vi "getHighlightedRows.vi"(8 "error in (no error)":errorcluster, 11 "OutcomeList in":refnum<class "GoalList.lvclass">) -> (0 "error out":errorcluster, 2 "Highlighted Rows":i32[](array[numeric]), 3 "OutcomeList out":refnum<class "GoalList.lvclass">)   [LabVIEW 2020, in "GoalList.lvclass"]
uses:
  GoalList.lvclass
  Goal/Goal.lvclass
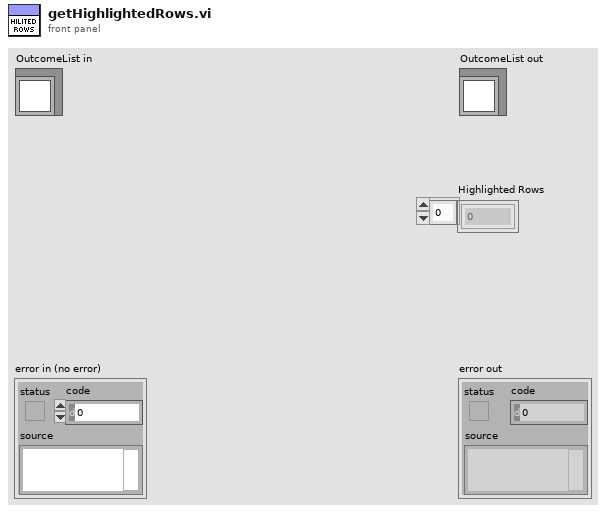
[diagram p1: front panel]
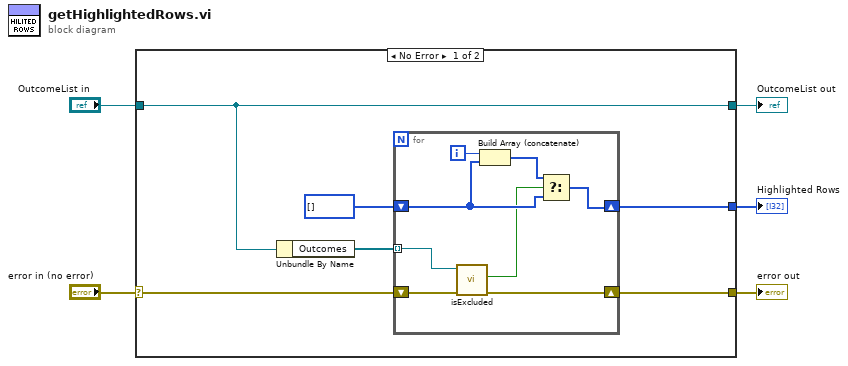
[diagram p0: block diagram]
diagram:
  n1 = case shown="No Error" "error in (no error)" {
    selector: "error in (no error)" -> [w8 w21]
    tunnel: [w7 w21] -> w4
    tunnel: [w9 w20] -> w2
    tunnel: "OutcomeList in" -> [w9 w20]
    tunnel: [w6 _] -> w1
    frame No Error {
      n2 = Unbundle By Name(w9) -> ("Outcomes"=w11:refnum<class "Goal.lvclass">[])
      n3 = for {
        tunnel: w11 -> [w15] mode=indexing
        shift-right: [w13] -> w7
        shift-left: w8 -> [w14]
        shift-right: [w19] -> w6
        shift-left: i32[] [] ("Highlighted Rows") -> [w17]
        i -> [w18]
        n4 = call "isExcluded.vi"("error in (no error)"=w14, "Goal in"=w15) -> ("error out"=w13:errorcluster, "Excluded?"=w12:bool)  [unwired: 7 in, 1 out]
        n5 = Build Array (concatenate)(w18, w17) -> (w16:i32[])
        n6 = Select(t=w16, s=w12, f=w17) -> (s? t:f=w19:i32[])
      }
    }
    frame Error {
    }
  }
  "error out" <- w4
  "OutcomeList out" <- w2
  "Highlighted Rows" <- w1
